vi "Convolution Example.vi"() -> ()   [LabVIEW 2012]
uses:
  User Controls/Array Dimensions.ctl
  Non-User VIs/Allocate Memory/AllocateMemory_32f.vi
  Non-User VIs/Write Memory/WriteMemory_32f.vi
  Non-User VIs/Read Memory/ReadMemory_32f.vi
  Non-User VIs/Error Checking/View Error Log Mode Functional Global.vi
  OpenCLV x64.lvlib
panel:
  in  "Kernel (5x5)":sgl[][][](array[numeric])=[[[0.0, 0.0, 1.0, 0.0, 0.0], [0.0, 1.0, -2.0, 1.0, 0.0], [1.0, -2.0, -6.0, -2.0, 1.0], [0.0, 1.0, -2.0, 1.0, 0.0], [0.0, 0.0, 1.0, 0.0, 0.0]]]
  out "Time in ms CPU":dbl
  out "Raw Image":sgl[][](graph)
  out "Processed Image":sgl[][](graph)
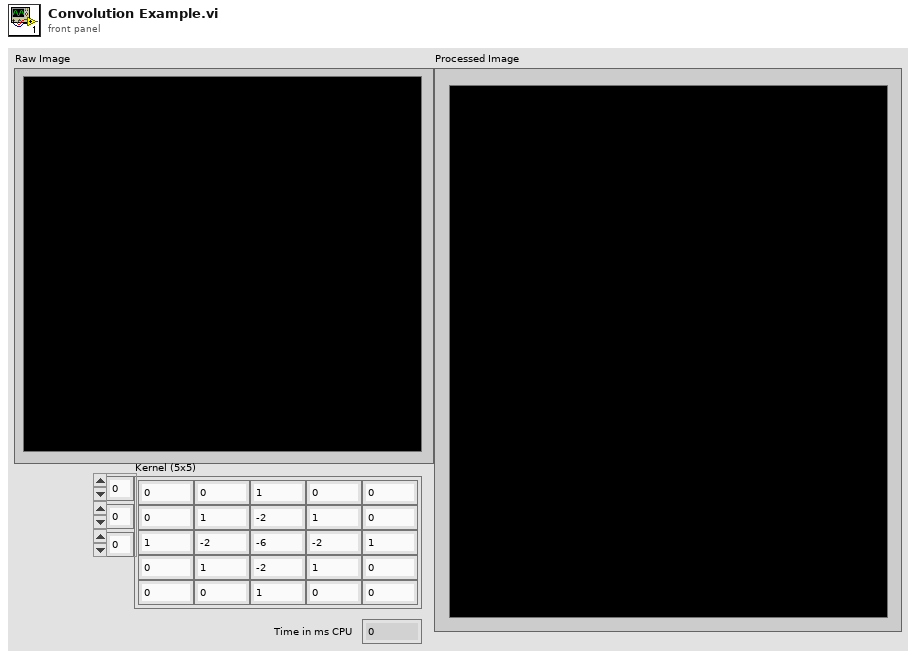
[diagram p1: front panel]
types:
  T1 = typedef "Array Dimensions.ctl" = cluster{"Depth":u64, "Height":u64, "Width":u64}
  T2 = typedef "imagedata.ctl" = cluster{"image type":i32, "image depth":i32, "image":u8[], "mask":u8[], "colors":u32[], "Rectangle":cluster{"left":i16, "top":i16, "right":i16, "bottom":i16}}
  T3 = typedef "OpenCLV x64.lvlib/Device ID.ctl" = u64
  T4 = typedef "OpenCLV x64.lvlib/Convolution Object.ctl" = cluster{"Device In":T3, "Program Handle":T5, "Kernel Memory Object":T6, "Convolved Memory Object":T6}
  T5 = typedef "OpenCLV x64.lvlib/Program Handle.ctl" = u64
  T6 = typedef "OpenCLV x64.lvlib/Memory Object.ctl" = cluster{"Device ID":T3, "Memeroy ID":T7, "Dimension":T1, "Memory Type":T8}
  T7 = typedef "OpenCLV x64.lvlib/Memory ID.ctl" = u64
  T8 = typedef "OpenCLV x64.lvlib/Memory Type.ctl" = enum16{"32f", "u8", "i8", "u16", "i16", "u32", "i32", "64f"}
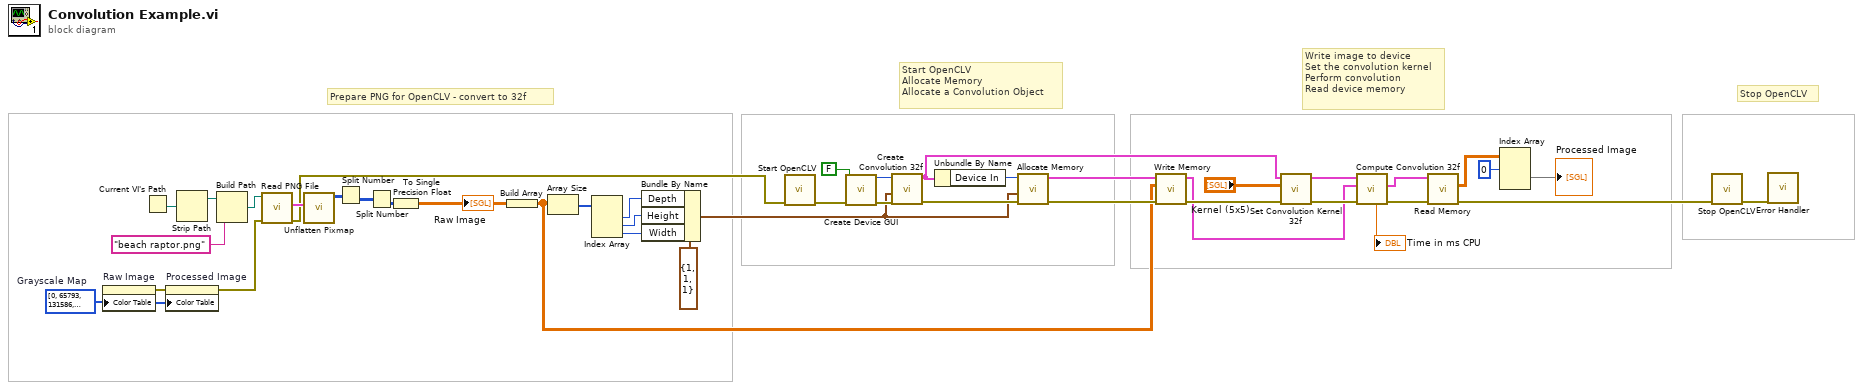
[diagram p0: block diagram]
diagram:
  w4 = u32[] [0, 65793, 131586, 197379, 263172, 328965, 394758, 460551, 526344, 592137, 657930, 723723, 789516, 855309, 921102, 986895, 1052688, 1118481, 1184274, 1250067, 1315860, 1381653, 1447446, 1513239, 1579032, 1644825, 1710618, 1776411, 1842204, 1907997, 1973790, 2039583, 2105376, 2171169, 2236962, 2302755, 2368548, 2434341, 2500134, 2565927, 2631720, 2697513, 2763306, 2829099, 2894892, 2960685, 3026478, 3092271, 3158064, 3223857, 3289650, 3355443, 3421236, 3487029, 3552822, 3618615, 3684408, 3750201, 3815994, 3881787, 3947580, 4013373, 4079166, 4144959, 4210752, 4276545, 4342338, 4408131, 4473924, 4539717, 4605510, 4671303, 4737096, 4802889, 4868682, 4934475, 5000268, 5066061, 5131854, 5197647, 5263440, 5329233, 5395026, 5460819, 5526612, 5592405, 5658198, 5723991, 5789784, 5855577, 5921370, 5987163, 6052956, 6118749, 6184542, 6250335, 6316128, 6381921, 6447714, 6513507, 6579300, 6645093, 6710886, 6776679, 6842472, 6908265, 6974058, 7039851, 7105644, 7171437, 7237230, 7303023, 7368816, 7434609, 7500402, 7566195, 7631988, 7697781, 7763574, 7829367, 7895160, 7960953, 8026746, 8092539, 8158332, 8224125, 8289918, 8355711, 8421504, 8487297, 8553090, 8618883, 8684676, 8750469, 8816262, 8882055, 8947848, 9013641, 9079434, 9145227, 9211020, 9276813, 9342606, 9408399, 9474192, 9539985, 9605778, 9671571, 9737364, 9803157, 9868950, 9934743, 10000536, 10066329, 10132122, 10197915, 10263708, 10329501, 10395294, 10461087, 10526880, 10592673, 10658466, 10724259, 10790052, 10855845, 10921638, 10987431, 11053224, 11119017, 11184810, 11250603, 11316396, 11382189, 11447982, 11513775, 11579568, 11645361, 11711154, 11776947, 11842740, 11908533, 11974326, 12040119, 12105912, 12171705, 12237498, 12303291, 12369084, 12434877, 12500670, 12566463, 12632256, 12698049, 12763842, 12829635, 12895428, 12961221, 13027014, 13092807, 13158600, 13224393, 13290186, 13355979, 13421772, 13487565, 13553358, 13619151, 13684944, 13750737, 13816530, 13882323, 13948116, 14013909, 14079702, 14145495, 14211288, 14277081, 14342874, 14408667, 14474460, 14540253, 14606046, 14671839, 14737632, 14803425, 14869218, 14935011, 15000804, 15066597, 15132390, 15198183, 15263976, 15329769, 15395562, 15461355, 15527148, 15592941, 15658734, 15724527, 15790320, 15856113, 15921906, 15987699, 16053492, 16119285, 16185078, 16250871, 16316664, 16382457, 16448250, 16514043, 16579836, 16645629, 16711422]  # Grayscale Map
  # "Stop OpenCLV"
  # "Write image to device\nSet the convolution kernel\nPerform convolution\nRead device memory"
  # "Start OpenCLV\nAllocate Memory\nAllocate a Convolution Object"
  # "Prepare PNG for OpenCLV - convert to 32f"
  n1 = property on="Raw Image" class="IntGraph (strict)"("Color Table"=w4) -> (error out=w5:errorcluster)  [unwired: 2 in, 1 out]
  n2 = Current VI's Path() -> (path=w42:path)
  n3 = property on="Processed Image" class="IntGraph (strict)"(error in=w5, "Color Table"=w4) -> (error out=w3:errorcluster)  [unwired: 1 in, 1 out]
  n4 = Strip Path(path=w42) -> (stripped path=w41:path)  [unwired: 1 out]
  n5 = Build Path(base path=w41, name or relative path="beach raptor.png") -> (appended path=w39:path)
  n6 = call <vilib>:"Read PNG File.vi"("error in (no error)"=w3, "path to PNG file"=w39) -> ("error out"=w2:errorcluster, "image data"=w38:T2)  [unwired: 7 in, 1 out]
  n7 = call <vilib>:"Unflatten Pixmap.vi"("image data"=w38) -> ("24-bit pixmap"=w37:u32[][])  [unwired: 4 in, 6 out]
  n8 = Split Number(x=w37) -> (lo(x)=w36:u16[][])  [unwired: 1 out]
  n9 = Split Number(x=w36) -> (lo(x)=w35:u8[][])  [unwired: 1 out]
  n10 = To Single Precision Float(number=w35) -> (single precision float=w13:sgl[][])
  "Raw Image" <- w13
  n11 = Build Array(w13) -> (w9:sgl[][][])
  n12 = Array Size(array=w9) -> (size(s)=w29:i32[])
  n13 = Index Array(array=w29) -> (element #1=w25:i32, element #2=w26:i32, element #3=w27:i32)  [unwired: 3 in]
  n14 = Bundle By Name(cluster=T1 {"Depth"=1, "Height"=1, "Width"=1} ("Dimension"), "Depth"=w25, "Height"=w26, "Width"=w27) -> (w12:T1)
  n15 = call "Start OpenCLV.vi"("Error In"=w2) -> ("Error Out"=w34:errorcluster)  [unwired: 10 in]
  n16 = call "Create Device GUI.vi"("Error In"=w34, "Skip Configuration"=FALSE) -> ("error constant"=w31:errorcluster, "Device Reference"=w32:T3)  [unwired: 8 in]
  n17 = call "Create Convolution 32f.vi"("Error In"=w31, "Convolution Dimensions"=w12, "Device In"=w32) -> ("Error Out"=w30:errorcluster, "Convolution Object"=w17:T4)  [unwired: 7 in]
  n18 = Unbundle By Name(w17) -> ("Device In"=w16:T3)
  n19 = call-poly "Allocate Memory.vi"("Error In"=w30, "Dimension"=w12, "Device In"=w16) -> ("Error Out"=w24:errorcluster, "Memory Object"=w20:T6)  [unwired: 6 in, 1 out]
  n20 = call-poly "Write Memory.vi"("Error In"=w24, "Data In"=w9, "Memory Object In"=w20) -> ("Error Out"=w21:errorcluster, "Memory Object Out"=w7:T6)  [unwired: 6 in, 1 out]
  n21 = call "Set Convolution Kernel 32f.vi"("Error In"=w21, "Kernel In"="Kernel (5x5)", "Convolution Object"=w17) -> ("Error Out"=w18:errorcluster, "Convolution Object Out"=w19:T4)  [unwired: 7 in]
  n22 = call "Compute Convolution 32f.vi"("Error In"=w18, "Input Memory"=w7, "Convolution Object"=w19) -> ("Error Out"=w23:errorcluster, "Convolved Memory"=w6:T6, "Time in ms"=→"Time in ms CPU":dbl)  [unwired: 5 in, 1 out]
  n23 = call-poly "Read Memory.vi"("Error In"=w23, "Memory Object In"=w6) -> ("Error Out"=w10:errorcluster, "Data Out"=w8:sgl[][][])  [unwired: 6 in, 2 out]
  n24 = Index Array(array=w8, index (dim 0)=0 ("index (page)")) -> (element=→"Processed Image":sgl[][])  [unwired: 2 in]
  n25 = call "Stop OpenCLV.vi"("Error In"=w10) -> ("Error Out"=w1:errorcluster)  [unwired: 10 in]
  n26 = call-poly "Error Handler.vi"("Error In"=w1) -> ()  [unwired: 10 in, 1 out]
